vi "Create Blank Save File.vi"(11 "Create Blank\nSave File":bool) -> ()   [LabVIEW 2016]
uses:
  <vilib>/Utility/file.llb/Write Delimited Spreadsheet (string).vi
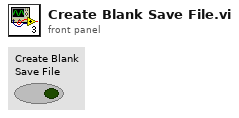
[diagram p1: front panel]
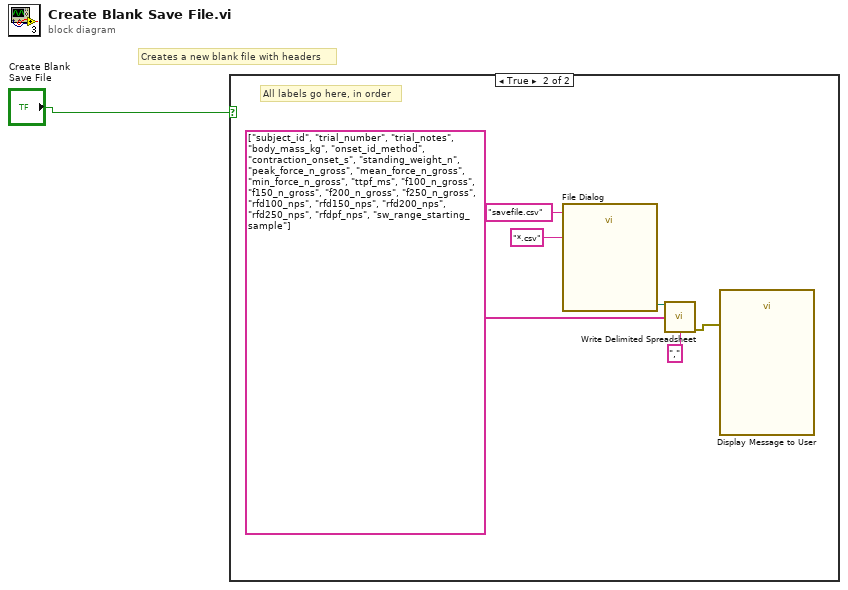
[diagram p0: block diagram]
diagram:
  # "Creates a new blank file with headers"
  n1 = case shown="True" "Create Blank\nSave File" {
    frame False {
    }
    frame True {
      # "All labels go here, in order"
      n2 = call "File Dialog"("default name"="savefile.csv", "pattern (all files)"="*.csv") -> ("selected path"=w4:path)  [unwired: 10 in, 3 out]
      n3 = call-poly <vilib>:"Write Delimited Spreadsheet.vi"("file path (dialog if empty)"=w4, "1D data"=string[] ["subject_id", "trial_number", "trial_notes", "body_mass_kg", "onset_id_method", "contraction_onset_s", "standing_weight_n", "peak_force_n_gross", "mean_force_n_gross", "min_force_n_gross", "ttpf_ms", "f100_n_gross", "f150_n_gross", "f200_n_gross", "f250_n_gross", "rfd100_nps", "rfd150_nps", "rfd200_nps", "rfd250_nps", "rfdpf_nps", "sw_range_starting_sample"], "delimiter (\\t)"="," ("delimiter (\\t)")) -> ("error out"=w6:errorcluster)  [unwired: 11 in, 1 out]
      n4 = call "Display Message to User"("error in (no error)"=w6) -> ()  [unwired: 9 in, 2 out]
    }
  }
